vi "Info from Folder.vi"(8 "error in (no error)":errorcluster, 9 "Name":string, 10 "Folder":path, 11 "Package in":refnum<class "Package.lvclass">) -> (0 "error out":errorcluster, 2 "Package Info":T1)   [LabVIEW 2020, in "GPack.lvlib" / "Package.lvclass"]
uses:
  Package.lvclass
  Package Info.ctl
  GPack.lvlib
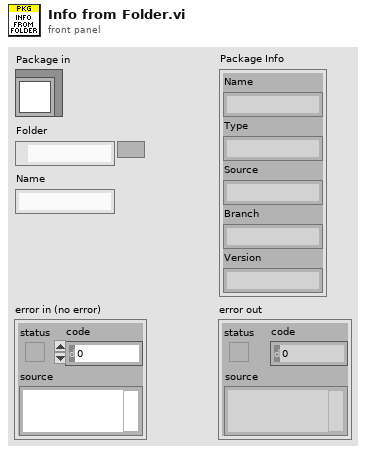
[diagram p1: front panel]
types:
  T1 = typedef "GPack.lvlib/Package Info.ctl" = cluster{"Name":string, "Type":string, "Source":string, "Branch":string, "Version":string}
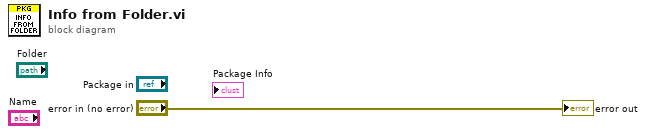
[diagram p0: block diagram]
diagram:
  "error out" <- "error in (no error)"
